vi "Log Event.vi"(8 "error in (no error)":errorcluster caption="错误输入（无错误）", 10 "事件文本":string, 11 "TPP demo V2 输入":refnum<class "TPP demo V2.lvclass">) -> (0 "error out":errorcluster caption="错误输出")   [LabVIEW 2017, in "TPP demo V2.lvlib" / "TPP demo V2.lvclass"]
uses:
  TPP demo V2.lvclass
  TPP demo V2.lvclass/TPP demo V2.ctl
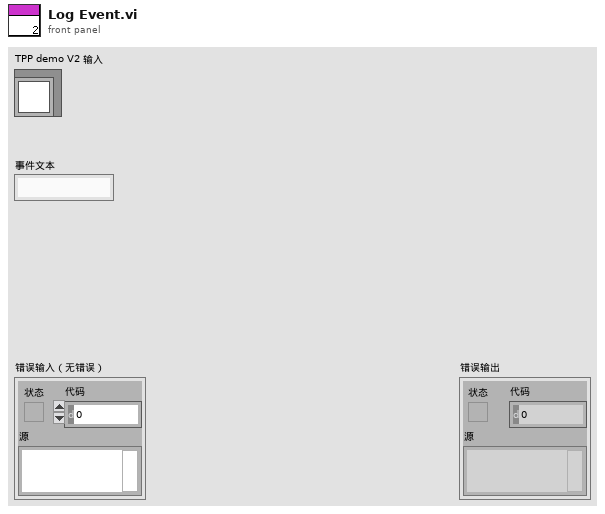
[diagram p1: front panel]
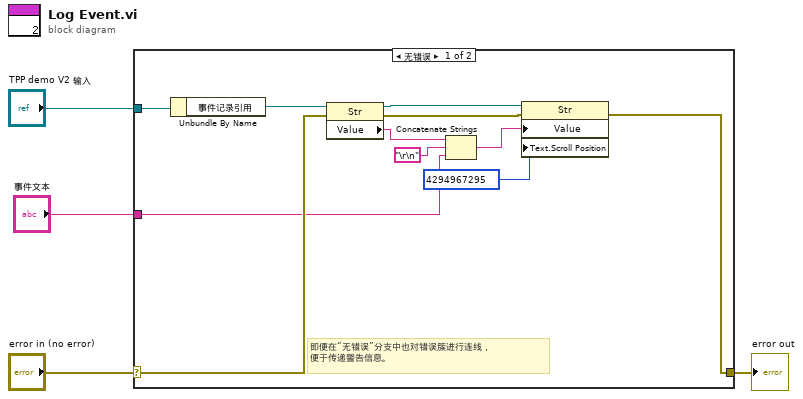
[diagram p0: block diagram]
diagram:
  n1 = case shown="无错误" "error in (no error)" {
    selector: "error in (no error)" -> [w13 w16]
    tunnel: [w5 w16] -> w3
    tunnel: "TPP demo V2 输入" -> [w15 _]
    tunnel: "事件文本" -> [w10 _]
    frame No Error {
      # "即便在“无错误”分支中也对错误簇进行连线，\n便于传递警告信息。"
      n2 = Unbundle By Name(w15) -> ("事件记录引用"=w14:refnum<vi>)
      n3 = property class="Str"(reference=w14, error in=w13) -> (reference out=w9:refnum<vi>, error out=w8:errorcluster, "Value"=w12:string)
      n4 = Concatenate Strings(w12, "\r\n", w10) -> (w7:string)
      n5 = property class="Str"(reference=w9, error in=w8, "Value"=w7, "Text.Scroll Position"=u32 4294967295 ("文本.滚动条位置")) -> (error out=w5:errorcluster)  [unwired: 1 out]
    }
    frame Error {
    }
  }
  "error out" <- w3
